vi "Prepare Aliases for UI.vi"(10 "Modules and Connections":T1[](array[typedef])=[{" Module Path"="", "Short Module Path"="", "Product Name"="", "Possible Connections"=[]}, {" Module Path"="", "Short Module Path"="", "Product Name"="", "Possible Connections"=[]}], 11 "Alias Mappings":T3[](array[typedef])) -> (2 "Mappings by Module UI":T5[](array[typedef]), 3 "Alias Mappings UI":T3[](array[typedef]))   [LabVIEW 2017, in "Routing and Faulting System Explorer.lvlib"]
uses:
  Routing and Faulting System Explorer.lvlib
  Shared/Alias Mapping.ctl
  Shared/Alias Endpoint.ctl
  Alias Map by Module.ctl
  Possible Connections.ctl
  Shared/Routing and Faulting Hardware API/Types/Possible Connections for Endpoint.ctl
  Shared/Routing and Faulting Shared.lvlib
  Shared/Routing and Faulting Hardware API/Routing and Faulting Hardware API.lvlib
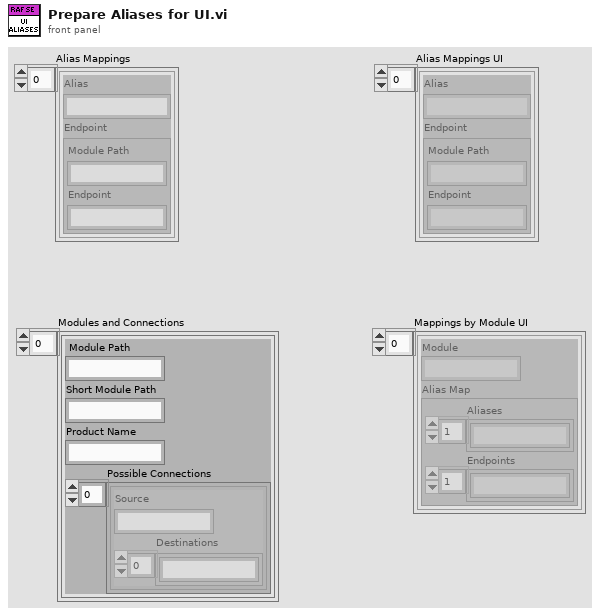
[diagram p1: front panel]
types:
  T1 = typedef "Routing and Faulting System Explorer.lvlib/Possible Connections.ctl" = cluster{" Module Path":string, "Short Module Path":string, "Product Name":string, "Possible Connections":T2[]}
  T2 = typedef "Routing and Faulting Hardware API.lvlib/Possible Connections for Endpoint.ctl" = cluster{"Source":string, "Destinations":string[]}
  T3 = typedef "Routing and Faulting Shared.lvlib/Alias Mapping.ctl" = cluster{"Alias":string, "Endpoint":T4}
  T4 = typedef "Routing and Faulting Shared.lvlib/Alias Endpoint.ctl" = cluster{"Module Path":string, "Endpoint":string}
  T5 = typedef "Routing and Faulting System Explorer.lvlib/Alias Map by Module.ctl" = cluster{"Module":string, "Alias Map":cluster{"Aliases":string[], "Endpoints":string[]}}
  T6 = cluster{"Module":string, "Alias Map":cluster{"Aliases":string[], "Endpoints":string[]}}
  T7 = cluster{"Module":string, "Alias Map":cluster{"Aliases":string[], "Endpoints":string[]}}[]
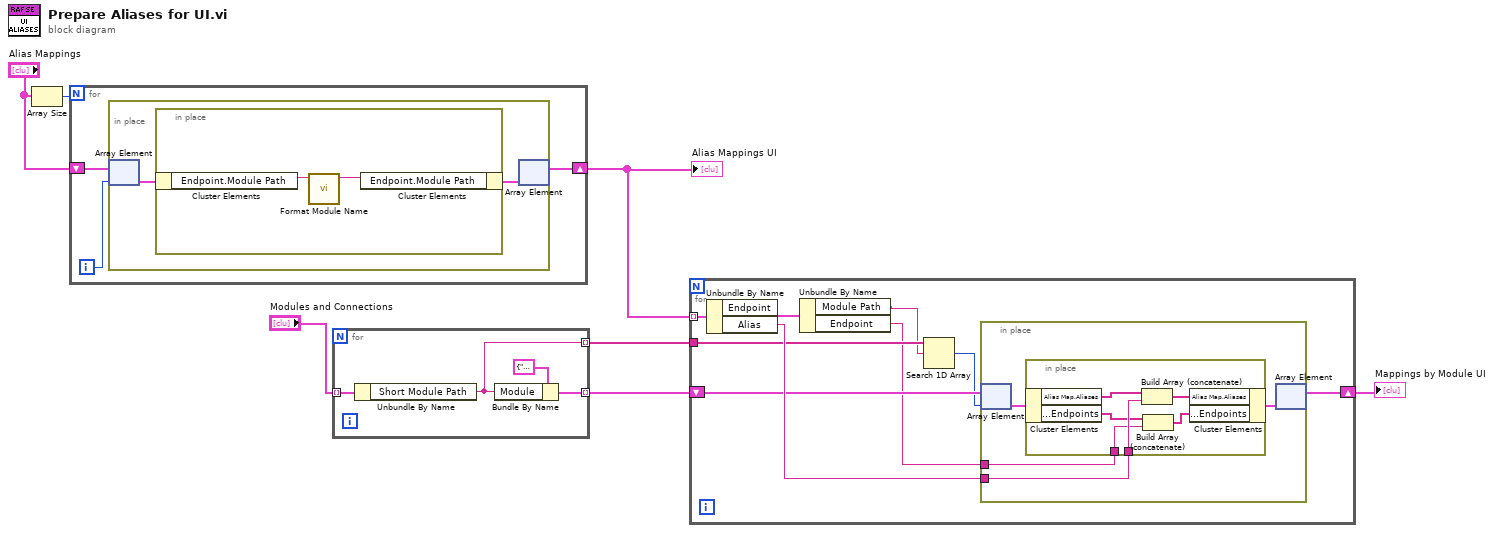
[diagram p0: block diagram]
diagram:
  n1 = Array Size(array="Alias Mappings") -> (size(s)=w6:i32)
  n2 = for {
    N: w6 -> [_]
    shift-right: [w8] -> w7
    shift-left: "Alias Mappings" -> [w10]
    i -> [w9]
    n3 = in-place {
      n4 = in-place-array #1(w10, w9) -> (w11:T3)
      n5 = in-place {
        n6 = in-place-cluster #2(w11) -> ("Endpoint.Module Path"=w13:string)
        n7 = call "Format Module Name.vi"("Module Path"=w13) -> ("Formatted Module Path"=w14:string)  [unwired: 10 in]
        n8 = in-place-cluster #2("Endpoint.Module Path"=w14) -> (w12:T3)
      }
      n9 = in-place-array #1(w12) -> (w8:T3[])  [unwired: 1 out]
    }
  }
  "Alias Mappings UI" <- w7
  n10 = for {
    tunnel: "Modules and Connections" -> [w18] mode=indexing
    tunnel: [w16] -> w2 mode=indexing
    tunnel: [w15] -> w1 mode=indexing
    n11 = Unbundle By Name(w18) -> ("Short Module Path"=w15:string)
    n12 = Bundle By Name(cluster=T6 {"Module"="", "Alias Map"={"Aliases"=[], "Endpoints"=[]}} ("Alias Mappings"), "Module"=w15) -> (w16:T6)
  }
  n13 = for {
    shift-right: [w23] -> w4
    shift-left: w2 -> [w24]
    tunnel: w7 -> [w27] mode=indexing
    tunnel: w1 -> [w25]
    n14 = Unbundle By Name(w27) -> ("Endpoint"=w21:T4, "Alias"=w26:string)
    n15 = Unbundle By Name(w21) -> ("Module Path"=w20:string, "Endpoint"=w19:string)
    n16 = Search 1D Array(1D array=w25, element=w20) -> (index of element=w22:i32)  [unwired: 1 in]
    n17 = in-place {
      in-place-border: w19 -> [w31]
      in-place-border: w26 -> [w30]
      n18 = in-place-array #3(w24, w22) -> (w29:T6)
      n19 = in-place {
        in-place-border: w30 -> [w35]
        in-place-border: w31 -> [w34]
        n20 = in-place-cluster #4(w29) -> ("Alias Map.Aliases"=w37:string[], "Alias Map.Endpoints"=w32:string[])
        n21 = Build Array (concatenate)(w37, w35) -> (w36:string[])
        n22 = Build Array (concatenate)(w32, w34) -> (w33:string[])
        n23 = in-place-cluster #4("Alias Map.Aliases"=w36, "Alias Map.Endpoints"=w33) -> (w28:T6)
      }
      n24 = in-place-array #3(w28) -> (w23:T7)  [unwired: 1 out]
    }
  }
  "Mappings by Module UI" <- w4
